vi "Lvi Subsystem Set Channel Option.vi"(1 "SetIEPE":bool, 4 "SetScaling":bool, 5 "Coupling":u32, 6 "CurrentSource":u32, 7 "SensorGain":dbl, 8 "error in (no error)":errorcluster, 9 "SensorOffset":dbl, 10 "Channel":u32, 11 "TaskRef":i32) -> (0 "error out":errorcluster, 2 "function return":u32(ring), 3 "TaskRef out":i32)   [LabVIEW 2022 SP3, in "DtLvLink.lvlib"]
doc: "Calls directly into the entry points of the DLL of the Data Acq SDK to specify the sensor gain and offset, and/or if IEPE inputs are supported, the excitation current source and input coupling type for a virtual analog channel of the specified task. This VI is used by the higher-level VIs, DtOLSetChanGain and DtOLSetChanIepeOptions."
uses:
  DtLvLink.lvlib
  <userlib>/LV-Link3/DtLvLink_64.dll
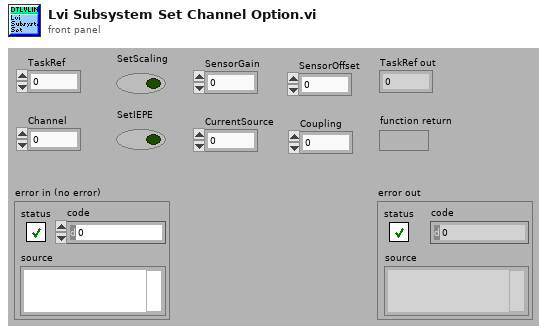
[diagram p1: front panel]
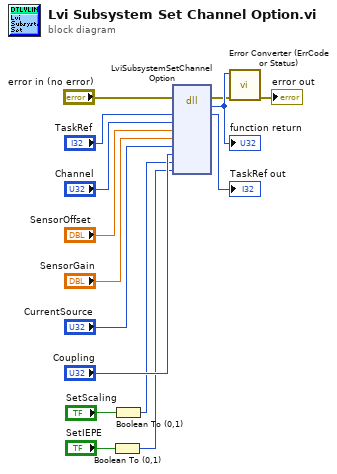
[diagram p0: block diagram]
diagram:
  n1 = Boolean To (0,1)(Boolean="SetIEPE") -> (0, 1=w1:i16)
  n2 = Boolean To (0,1)(Boolean="SetScaling") -> (0, 1=w2:i16)
  n3 = dll-call lib="C:/Program Files/National Instruments/LabVIEW 2022/user.lib/LV-Link3/DtLvLink_64.*" fn="LviSubsystemSetChannelOption"(error in="error in (no error)", "TaskRef"="TaskRef", "Channel"="Channel", "SensorOffset"="SensorOffset", "SensorGain"="SensorGain", "CurrentSource"="CurrentSource", "Coupling"="Coupling", "SetScaling"=w2, "SetIEPE"=w1) -> (error out=w6:errorcluster, "return type"=w15:u32, "TaskRef"=→"TaskRef out":i32)  [unwired: 9 in, 1 out]
  "function return" <- w15
  n4 = call "Error Converter (ErrCode or Status).vi"("error in (no error)"=w6, "error code"=w15) -> ("error out"=→"error out":errorcluster)  [unwired: 9 in]
